vi "SPI Init Channel.vi"(8 "error in (no error)":errorcluster, 10 "config":T1={"ClockRate"=5000, "LatencyTimer"=30, "configOptions 0-7"=0, "configOptions 8-15"=0, "configOptions 16-23"=0, "configOptions 24-31"=0, "Pin"=0, "reserved"=0}, 11 "handle":u32 format="%08x") -> (0 "error out":errorcluster, 3 "handle out":u32 format="%08x")   [LabVIEW 2018, in "libMPSSE-SPI.lvlib"]
doc: "FTDI_API FT_STATUS SPI_InitChannel(FT_HANDLE handle, ChannelConfig *config);"
uses:
  libMPSSE-SPI.lvlib
  dll/libMPSSE.dll
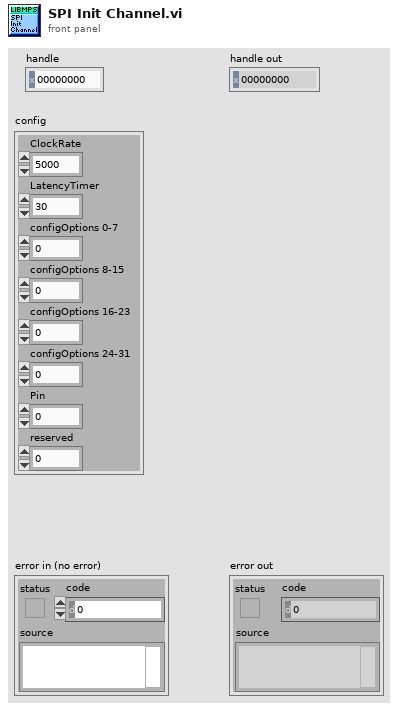
[diagram p1: front panel]
types:
  T1 = cluster{"ClockRate":u32, "LatencyTimer":u8, "configOptions 0-7":i8, "configOptions 8-15":i8, "configOptions 16-23":i8, "configOptions 24-31":u32, "Pin":u32, "reserved":u16}
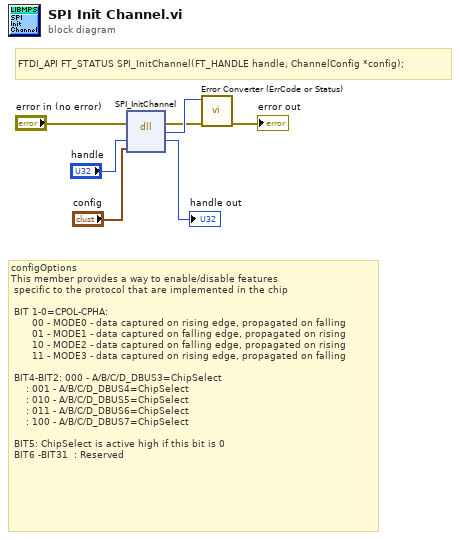
[diagram p0: block diagram]
diagram:
  # "configOptions\nThis member provides a way to enable/disable features\n\tspecific to the protocol that are implemented in the chip\n\n\tBIT 1-0=CPOL-CPHA:\t\n       00 - MODE0 - data captured on rising edge, propagated on falling\n \t\t\t\t\t\t01 - MODE1 - data captured on falling edge, propagated on rising\n \t\t\t\t\t\t10 - MODE2 - data captured on falling edge, propagated on rising\n \t\t\t\t\t\t11 - MODE3 - data captured on rising edge, propagated on falling\n\n\tBIT4-BIT2: 000 - A/B/C/D_DBUS3=ChipSelect\n\t\t\t  : 001 - A/B/C/D_DBUS4=ChipSelect\n \t\t\t : 010 - A/B/C/D_DBUS5=ChipSelect\n \t\t\t : 011 - A/B/C/D_DBUS6=ChipSelect\n \t\t\t : 100 - A/B/C/D_DBUS7=ChipSelect\n\n BIT5: ChipSelect is active high if this bit is 0\n\tBIT6 -BIT31\t\t: Reserved"
  # "FTDI_API FT_STATUS SPI_InitChannel(FT_HANDLE handle, ChannelConfig *config);"
  n1 = dll-call lib="D:/LABVIEW/Examples - 32bit/FTDI/libMPSSE-SPI-LabVIEW-master/dll/libMPSSE.*" fn="SPI_InitChannel"(error in="error in (no error)", "handle"="handle", "config"="config") -> (error out=w2:errorcluster, "return type"=w7:u32, "handle"=→"handle out":u32)  [unwired: 3 in, 1 out]
  n2 = call "Error Converter (ErrCode or Status).vi"("error in (no error)"=w2, "error code"=w7) -> ("error out"=→"error out":errorcluster)  [unwired: 9 in]
